vi "MGI Read Key (String[]).vi"(7 "Section":string, 8 "error in (no error)":errorcluster, 9 "Default Value[]":string[](array[string]), 10 "Key":string, 11 "Refnum":T1) -> (0 "error out":errorcluster, 1 "Value[]":string[](array[string]), 2 "Found?":bool, 3 "Refnum":T1)   [LabVIEW 2016]
doc: "Read a 1D string array key (actually a section) written by the matching Write VI.\n\nFreeware from Moore Good Ideas, www.mooregoodideas.com. Do not remove this line."
uses:
  <vilib>/Utility/config.llb/Config Data RefNum.ctl
  <vilib>/Utility/config.llb/Read Key (I32).vi
  <vilib>/Utility/config.llb/Read Key (String).vi
  <vilib>/Utility/config.llb/NI_LVConfig.lvlib
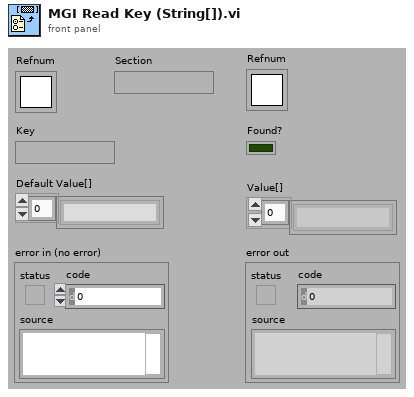
[diagram p1: front panel]
types:
  T1 = typedef "NI_LVConfig.lvlib/Config Data RefNum.ctl" = refnum<k1>
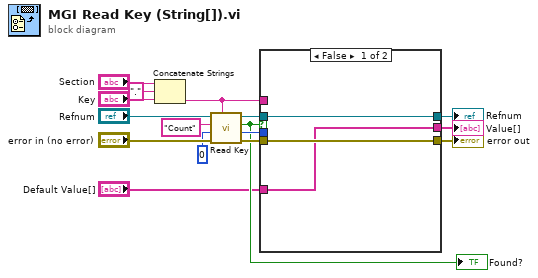
[diagram p0: block diagram]
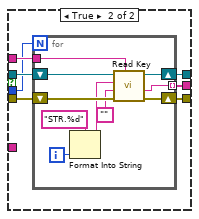
[diagram p2: hidden frame]
diagram:
  n1 = Concatenate Strings("Section", "." ("Substring"), "Key") -> (w8:string)
  n2 = call-poly <vilib>:"Read Key.vi"("section"=w8, "error in (no error)"="error in (no error)", "default value"=0, "key"="Count", "refnum"="Refnum") -> ("error out"=w15:errorcluster, "value"=w4:i32, "found?"=w2:bool, "refnum out"=w14:T1)  [unwired: 3 in]
  "Found?" <- w2
  n3 = case shown="False" w2 {
    tunnel: w15 -> [w18 w26]
    tunnel: w14 -> [w19 w25]
    tunnel: [w18 w24] -> w13
    tunnel: [w19 w23] -> w12
    tunnel: w8 -> [_ w22]
    tunnel: w4 -> [_ w21]
    tunnel: [w17 w20] -> w3
    tunnel: "Default Value[]" -> [w17 _]
    frame False {
    }
    frame True {
      n4 = for {
        N: w21 -> [_]
        shift-right: [w33] -> w24
        shift-left: w26 -> [w36]
        shift-right: [w32] -> w23
        shift-left: w25 -> [w35]
        tunnel: w22 -> [w34]
        tunnel: [w27] -> w20 mode=indexing
        i -> [w31]
        n5 = Format Into String(format string="STR.%d" ("Format String"), w31) -> (resulting string=w30:string)  [unwired: 2 in, 1 out]
        n6 = call-poly <vilib>:"Read Key.vi"("section"=w34, "error in (no error)"=w36, "default value"="", "key"=w30, "refnum"=w35) -> ("error out"=w33:errorcluster, "value"=w27:string, "refnum out"=w32:T1)  [unwired: 3 in, 1 out]
      }
    }
  }
  "Value[]" <- w3
  "error out" <- w13
  "Refnum" <- w12
